vi "Timer global variable.vi"() -> ()   [LabVIEW 2021, in "Named Timers.lvlib"]
uses:
  Named Timers.lvlib
  Timer Cluster.ctl
panel:
  in  "Timers":T1[](array[typedef])
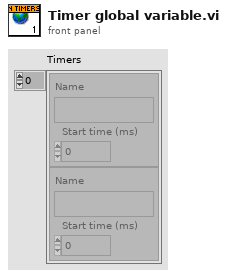
[diagram p1: front panel]
types:
  T1 = typedef "Named Timers.lvlib/Timer Cluster.ctl" = cluster{"Name":string, "Start time (ms)":u32}
diagram:
